vi "WPI_UtilitiesFRCAutomaticValuePublisherImpl.vi"(11 "Enable":bool=TRUE) -> ()   [LabVIEW 2025]
uses:
  <vilib>/Rock Robotics/WPI/Utilities/Refnum Registry Operation.ctl
  <vilib>/Rock Robotics/WPI/Relay/WPI_RelayValue.ctl
  <vilib>/Rock Robotics/WPI/Solenoid/WPI_SolenoidValue.ctl
  <vilib>/Rock Robotics/WPI/Solenoid/WPI_SolenoidChannel.ctl
  <vilib>/Rock Robotics/WPI/Solenoid/WPI_SolenoidSetEnum.vi
  <vilib>/Rock Robotics/WPI/Ultrasonic/WPI_SonarSRF04DigitalRefNum Registry Get.vi
  <vilib>/Rock Robotics/WPI/Ultrasonic/WPI_SonarSRF04DigitalGetRange.vi
  <vilib>/Rock Robotics/WPI/Ultrasonic/WPI_SonarSRF08_I2C_RefNum Registry Get.vi
  <vilib>/Rock Robotics/WPI/Ultrasonic/WPI_SonarSRF08_I2C_GetRange.vi
  <vilib>/Rock Robotics/WPI/Ultrasonic/WPI_SonarMB1010DigitalRefNum Registry Get.vi
  <vilib>/Rock Robotics/WPI/Ultrasonic/WPI_SonarMB1010DigitalGetRange.vi
  <vilib>/Rock Robotics/WPI/Ultrasonic/WPI_SonarMB1010AnalogRefNum Registry Get.vi
  <vilib>/Rock Robotics/WPI/Ultrasonic/WPI_SonarMB1010AnalogGetRange.vi
  <vilib>/Rock Robotics/Network Tables/NT Write Integer.vi
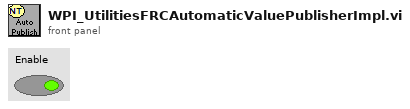
[diagram p1: front panel]
types:
  T1 = typedef "Refnum Registry Operation.ctl" = enum16{"set", "get", "delete", "get all names", "read name"}
  T2 = typedef "WPI_RelayValue.ctl" = enum16{"Off", "On", "Forward", "Reverse"}
  T3 = typedef "WPI_SolenoidChannel.ctl" = enum8{"Solenoid 0", "Solenoid 1", "Solenoid 2", "Solenoid 3", "Solenoid 4", "Solenoid 5", "Solenoid 6", "Solenoid 7", "Solenoid 8", "Solenoid 9", "Solenoid 10", "Solenoid 11", "Solenoid 12", "Solenoid 13", "Solenoid 14", "Solenoid 15", "Invalid"}
  T4 = typedef "WPI_SolenoidValue.ctl" = enum16{"Off", "On", "Forward", "Reverse"}
  T5 = enum16{"None", "XON/XOFF", "RTS/CTS", "XON/XOFF & RTS/CTS", "DTR/DSR", "XON/XOFF & DTR/DSR"}
  T6 = typedef "WPI_JoystickDevRef.ctl" = cluster{"Device":T7}
  T7 = typedef "WPI_JoystickDeviceEnum.ctl" = enum16{"USB 0", "USB 1", "USB 2", "USB 3", "USB 4", "USB 5"}
  T8 = typedef "WPI_Joystick Info.ctl" = cluster{"Device Name":string, "HID Type":T9, "XBox Type":T10, "Axes Count":i32, "Axes Types":T11[], "Button Count":i32, "POV Count":i32}
  T9 = typedef "WPI_JoystickHID Types.ctl" = enum16{"Not HID", "HID Joystick", "HID Gamepad", "HID Driving Wheel", "HID Flightstick", "HID First Person"}
  T10 = typedef "WPI_JoystickXBox Types.ctl" = enum16{"Not XBox", "XBox Unknown", "XBox Gamepad", "XBox Wheel", "XBox Arcade Stick", "XBox Flight Stick", "XBox Dance Pad", "XBox Guitar", "XBox Drum Kit", "XBox Arcade Pad"}
  T11 = typedef "WPI_JoystickAxis Types.ctl" = enum16{"X Axis", "Y Axis", "Z Axis", "RxAxis", "RyAxis", "RzAxis", "Slider", "POV", "None", "L X Axis", "L Y Axis", "L Trigger", "R Trigger", "R X Axis", "R Y Axis"}
  T12 = typedef "WPI_MotorControlDeviceRef.ctl" = cluster{"DeviceStatus":errorcluster, "Type":T13, "PWM":cluster{"PWM Channel":T14, "DeadBand":T15}, "CAN":cluster{"Device Number":u8, "SetOutput VI Ref":variant, "GetOutput VI Ref":variant, "Enable VI Ref":variant, "Disable VI Ref":variant, "Data":variant}, "Invert":bool, "DIO PWM":cluster{"PWM \"Enable\" Channel":T14, "DIOChannel":T16, "PWM Rate":dbl}}
  T13 = typedef "WPI_MotorControlType.ctl" = enum16{"PWM", "CAN", "DIO PWM"}
  T14 = typedef "FPGA_DIOPWMChannel.ctl" = enum8{"PWM 0", "PWM 1", "PWM 2", "PWM 3", "PWM 4", "PWM 5", "PWM 6", "PWM 7", "PWM 8", "PWM 9", "PWM MXP 0", "PWM MXP 1", "PWM MXP 2", "PWM MXP 3", "PWM MXP 4", "PWM MXP 5", "PWM MXP 6", "PWM MXP 7", "PWM MXP 8", "PWM MXP 9", "Invalid"}
  T15 = typedef "WPI_PWMDeadband.ctl" = cluster{"Name":string, "maxPositivePwm":i32, "minPositivePwm":i32, "centerPwm":i32, "maxNegativePwm":i32, "minNegativePwm":i32, "angularRange":u16}
  T16 = typedef "FPGA_DIOChannel.ctl" = enum8{"DIO 0", "DIO 1", "DIO 2", "DIO 3", "DIO 4", "DIO 5", "DIO 6", "DIO 7", "DIO 8", "DIO 9", "DIO MXP 0", "DIO MXP 1", "DIO MXP 2", "DIO MXP 3", "DIO MXP 4", "DIO MXP 5", "DIO MXP 6", "DIO MXP 7", "DIO MXP 8", "DIO MXP 9", "DIO MXP 10", "DIO MXP 11", "DIO MXP 12", "DIO MXP 13", "DIO MXP 14", "DIO MXP 15", "SPI Port CS1", "SPI Port CS2", "SPI Port CS3", "SPI Port MISO", "SPI Port MOSI", "Invalid"}
  T17 = typedef "WPI_ServoDeviceRef.ctl" = cluster{"DeviceStatus":errorcluster, "PWM Channel":T14, "DeadBand":T15}
  T18 = typedef "WPI_RelayDevRef.ctl" = cluster{"DevStatus":errorcluster, "Relay Channel":T19, "Relay Direction":T20}
  T19 = typedef "FPGA_DIORelayChannel.ctl" = enum8{"Relay 0", "Relay 1", "Relay 2", "Relay 3", "Invalid"}
  T20 = typedef "WPI_RelayDirection.ctl" = enum16{"Both directions", "Forward only", "Reverse only"}
  T21 = typedef "WPI_CompressorDevRef.ctl" = cluster{"DevStatus":errorcluster, "Pneumatics Control Module":u8}
  T22 = typedef "WPI_SolenoidDevRef.ctl" = cluster{"DevStatus":errorcluster, "Pneumatics Control Module":u8, "Forward Solenoid Channel":T3, "Reverse Solenoid Channel":T3}
  T23 = typedef "WPI_AccelerometerDevRef.ctl" = cluster{"DevStatus":errorcluster, "Scaling":T24, "Analog Channels":T25, "I2C Bus":T27, "SPI Bus":T28, "Accel Range":T29, "ADXL Axes":T30, "Handle":i32, "Device Address":u8, "Accel Type":enum16{"Analog", "ADXL345 I2C", "ADXL345 SPI", "Internal", "ADXL362 SPI"}}
  T24 = typedef "WPI_AccelerometerScaling.ctl" = cluster{"Gain (VoltsPerG)":dbl, "Center Voltage":dbl}
  T25 = typedef "WPI_AccelerometerAnalogChannels.ctl" = cluster{"X-Axis":T26, "Y-Axis":T26, "Z-Axis":T26}
  T26 = typedef "FPGA_AIChannel.ctl" = enum8{"AI 0", "AI 1", "AI 2", "AI 3", "AI MXP 0", "AI MXP 1", "AI MXP 2", "AI MXP 3", "Invalid"}
  T27 = typedef "i2c_bus.ctl" = enum16{"I2C On-Board", "I2C MXP", "Invalid"}
  T28 = typedef "spi_bus.ctl" = enum16{"SPI On-Board, CS0", "SPI On-Board, CS1", "SPI On-Board, CS2", "SPI On-Board, CS3", "SPI MXP", "Invalid"}
  T29 = typedef "ADXL345 Range.ctl" = u8
  T30 = typedef "WPI_AccelerometerADXL345 Axes.ctl" = cluster{"X-Axis":bool, "Y-Axis":bool, "Z-Axis":bool}
  T31 = cluster{"X-Axis":dbl, "Y-Axis":dbl, "Z-Axis":dbl}
  T32 = typedef "WPI_CounterDevRef.ctl" = cluster{"DevStatus":errorcluster, "CntIndex":T33}
  T33 = typedef "FPGA_CounterCtrSystemIndex.ctl" = enum8{"Ctr 0", "Ctr 1", "Ctr 2", "Ctr 3", "Ctr 4", "Ctr 5", "Ctr 6", "Ctr 7", "Invalid"}
  T34 = typedef "WPI_GyroDevRef.ctl" = cluster{"DevStatus":errorcluster, "Analog Channel":T26, "Gain (VoltsPerDegree/Second)":dbl, "Gyro Type":enum16{"Analog", "XRS450"}, "Handle":i32, "SPI Bus":T28, "Device Found":bool, "Sample Rate":dbl, "Calibrate On Open":bool, "Offset":dbl}
  T35 = typedef "WPI_UltrasonicDeviceRef.ctl" = cluster{"DevStatus":errorcluster, "Ping Channel":T16, "Echo Channel":T16, "CntIndex":T33}
  T36 = typedef "WPI_SonarSRF08_I2C_DeviceRef.ctl" = cluster{"I2CDevRef":T37}
  T37 = typedef "WPI_I2CDevRef.ctl" = cluster{"DevStatus":errorcluster, "Device Address":u8, "Handle":i32, "I2C Bus":T27}
  T38 = typedef "WPI_SonarMB1010DigitalDeviceRef.ctl" = cluster{"CounterDevRef":T32, "Scaling factor (s/in)":dbl}
  T39 = typedef "WPI_SonarMB1010AnalogDeviceRef.ctl" = cluster{"AIDeviceRef":T40, "Scaling factor (V/in)":dbl, "Average Bits":u8}
  T40 = typedef "WPI_AnalogChannelDevRef.ctl" = cluster{"DevStatus":errorcluster, "Analog Channel":T26}
  T41 = typedef "WPI_DigitalInputDevRef.ctl" = cluster{"DevStatus":errorcluster, "DIO Channel":T16}
  T42 = typedef "WPI_SwitchDevRef.ctl" = cluster{"DevStatus":errorcluster, "DIO Channel":T16, "CntIndex":T33, "Normally Closed":bool}
  T43 = typedef "WPI_EncoderDevRef.ctl" = cluster{"DevStatus":errorcluster, "EncoderIndex":T44, "CounterIndex":T33, "DistancePerCount":dbl, "Decoding Type":T45}
  T44 = typedef "FPGA_EncoderIdx.ctl" = enum8{"Enc 0", "Enc 1", "Enc 2", "Enc 3", "Enc 4", "Enc 5", "Enc 6", "Enc 7", "Invalid"}
  T45 = typedef "WPI_EncoderType.ctl" = enum16{"1x", "2x", "4x"}
  T46 = typedef "WPI_DigitalOutputDevRef.ctl" = cluster{"DIO Channel":T16, "DevStatus":errorcluster}
  T47 = typedef "WPI_AOChannelDevRef.ctl" = cluster{"DevStatus":errorcluster, "AO Channel":T48}
  T48 = typedef "WPI_AnalogOutputChannel.ctl" = enum8{"AO MXP 0", "AO MXP 1", "Invalid"}
  T49 = typedef "WPI_PWMDeviceRef.ctl" = cluster{"DeviceStatus":errorcluster, "PWM Channel":T14}
  T50 = typedef "WPI_PotentiometerDevRef.ctl" = cluster{"DevStatus":errorcluster, "Analog Channel":T26, "Invert Output":bool}
  T51 = typedef "WPI_CameraDevRef.ctl" = cluster{"Camera Address":string, "CameraStatus":errorcluster}
  T52 = typedef "WPI_SerialPortRef.ctl" = cluster{"DevStatus":errorcluster, "Serial Port Name":refnum<visa-resource-name>}
  T53 = typedef "WPI_SPIDevRef.ctl" = cluster{"DevStatus":errorcluster, "Handle":i32, "SPI Bus":T28}
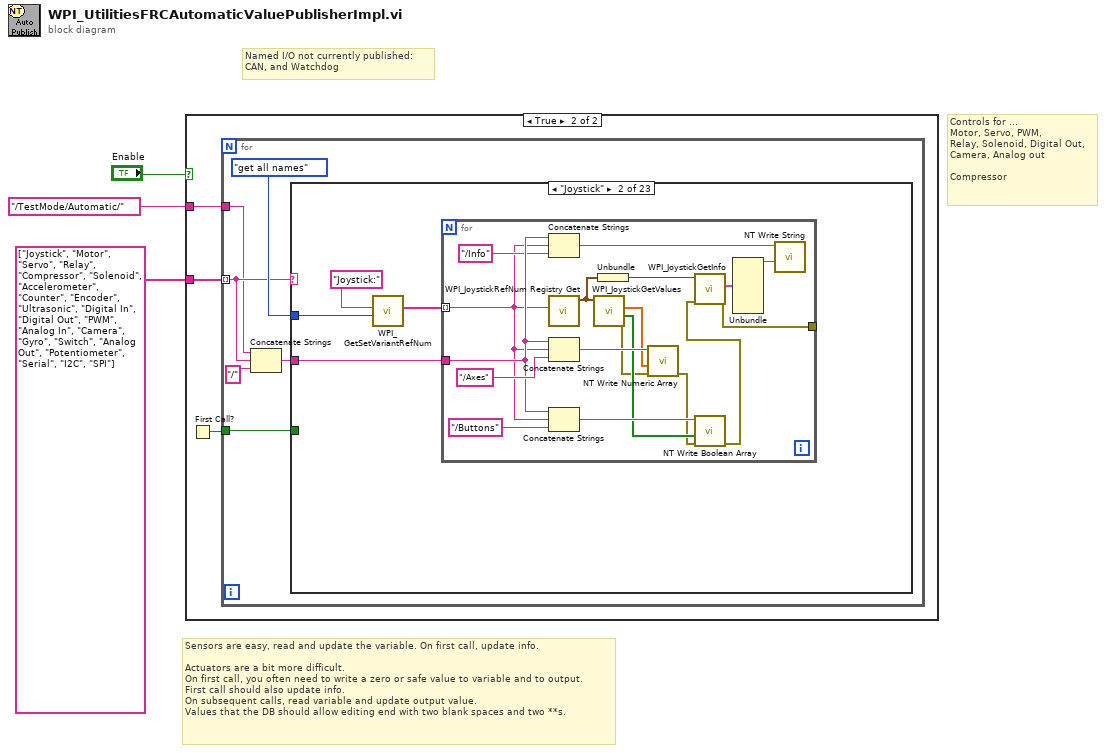
[diagram p0: block diagram]
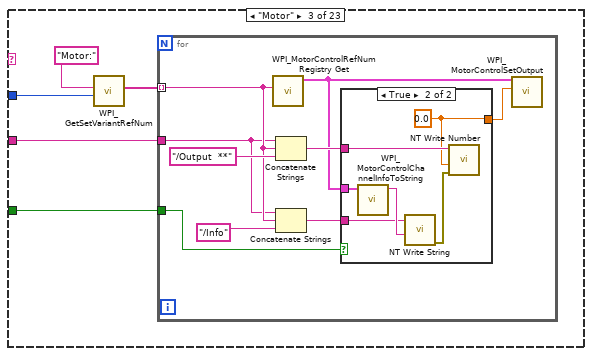
[diagram p4: hidden frame]
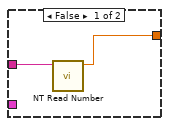
[diagram p5: hidden frame]
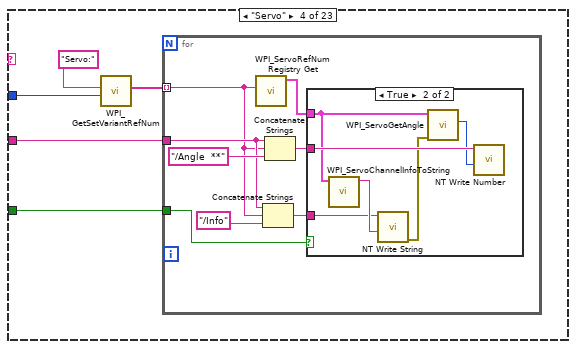
[diagram p6: hidden frame]
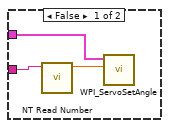
[diagram p7: hidden frame]
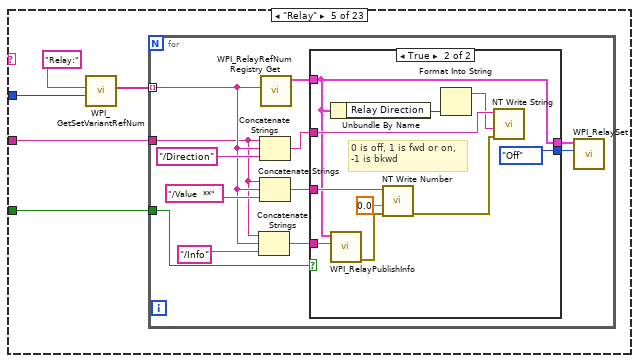
[diagram p8: hidden frame]
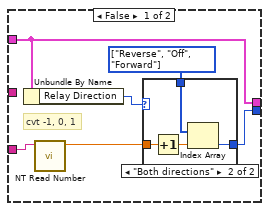
[diagram p9: hidden frame]
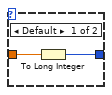
[diagram p10: hidden frame]
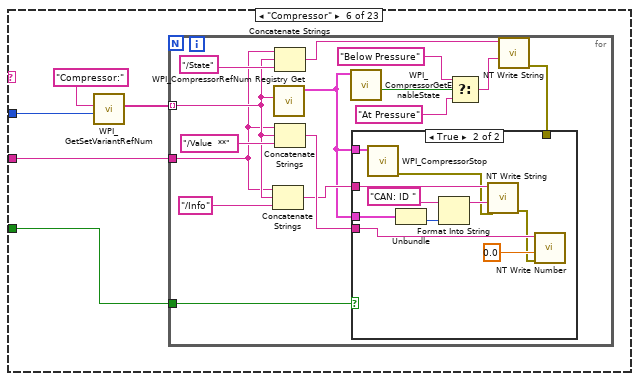
[diagram p11: hidden frame]
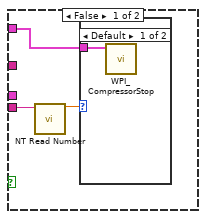
[diagram p12: hidden frame]
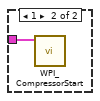
[diagram p13: hidden frame]
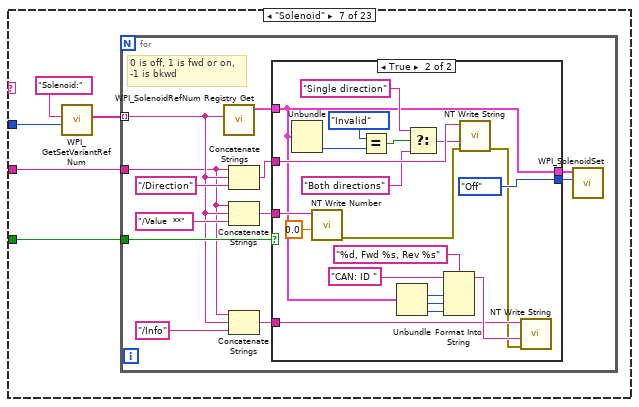
[diagram p14: hidden frame]
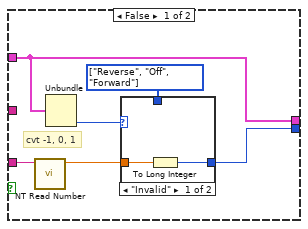
[diagram p15: hidden frame]
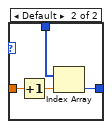
[diagram p16: hidden frame]
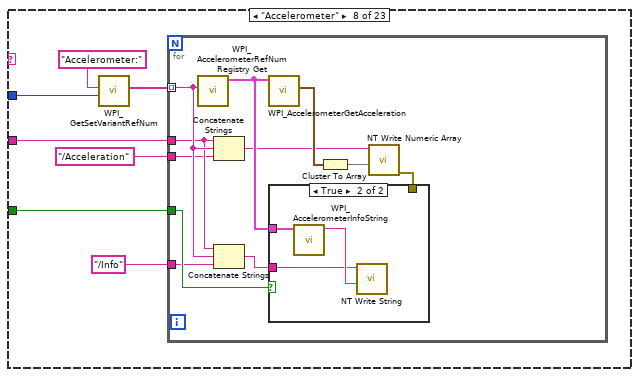
[diagram p17: hidden frame]
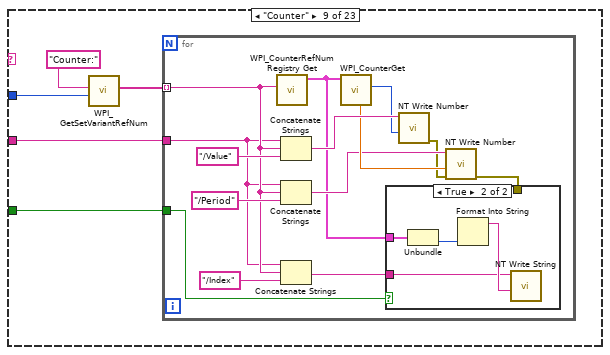
[diagram p19: hidden frame]
diagram:
  # "Controls for ...\nMotor, Servo, PWM,\nRelay, Solenoid, Digital Out,\nCamera, Analog out\n\nCompressor"
  # "Named I/O not currently published:\nCAN, and Watchdog"
  # "Sensors are easy, read and update the variable. On first call, update info.\n\nActuators are a bit more difficult. \nOn first call, you often need to write a zero or safe value to variable and to output.\nFirst call should also update info.\nOn subsequent calls, read variable and update output value.\nValues that the DB should allow editing end with two blank spaces and two **s."
  n1 = case shown="True" "Enable" {
    tunnel: string[] ["Joystick", "Motor", "Servo", "Relay", "Compressor", "Solenoid", "Accelerometer", "Counter", "Encoder", "Ultrasonic", "Digital In", "Digital Out", "PWM", "Analog In", "Camera", "Gyro", "Switch", "Analog Out", "Potentiometer", "Serial", "I2C", "SPI"] -> [_ w6]
    tunnel: "/TestMode/Automatic/" -> [_ w4]
    frame False {
    }
    frame True {
      n2 = First Call?() -> (First Call?: T/F=w5:bool)
      n3 = for {
        tunnel: w6 -> [w10] mode=indexing
        tunnel: w5 -> [w11]
        tunnel: w4 -> [w9]
        n4 = Concatenate Strings(w9, w10, "/") -> (w7:string)
        n5 = case shown="\"Joystick\"" w10 {
          tunnel: Refnum_Registry_Operation."get all names" ("menu") -> [_ w14 w36 w57 w79 w119 w153 w204 w223 w246 w271 w358 w375 w400 w426 w453 w479 w503 w523 w547 w569 w602 w618]
          tunnel: w11 -> [_ _ w39 w61 w83 w122 w157 w208 w227 w250 w273 w362 w379 w404 w430 w457 w483 w507 w527 w551 w568 w601 w617]
          tunnel: w7 -> [_ w16 w38 w60 w82 w121 w156 w207 w226 w249 w272 w361 w378 w403 w429 w456 w482 w506 w526 w550 w570 w603 w619]
          frame Default {
            # "Unsupported I/O type"
          }
          frame "Joystick" {
            n6 = call <vilib>:"WPI_GetSetVariantRefNum.vi"("Operation"=w14, "refnum name"="Joystick:") -> ("names"=w15:string[])  [unwired: 7 in, 2 out]
            n7 = for {
              tunnel: w15 -> [w23] mode=indexing
              tunnel: w16 -> [w25]
              tunnel: [w19] -> _
              n8 = Concatenate Strings(w25, w23, "/Info") -> (w18:string)
              n9 = call <vilib>:"WPI_JoystickRefNum Registry Get.vi"("refnum name"=w23) -> ("JoystickDevRef"=w28:T6)  [unwired: 9 in, 1 out]
              n10 = Concatenate Strings(w25, w23, "/Axes") -> (w31:string)
              n11 = Concatenate Strings(w25, w23, "/Buttons") -> (w33:string)
              n12 = call <vilib>:"WPI_JoystickGetValues.vi"("JoystickDevRef"=w28) -> ("error out"=w20:errorcluster, "Buttons"=w29:bool[], "Axes"=w30:dbl[])  [unwired: 6 in, 2 out]
              n13 = Unbundle(w28) -> ("Device"=w27:T7)
              n14 = call <vilib>:"NT Write Numeric Array.vi"("error in"=w20, "value"=w30, "name"=w31) -> ("error out"=w22:errorcluster)  [unwired: 8 in]
              n15 = call <vilib>:"NT Write Boolean Array.vi"("error in"=w22, "value"=w29, "name"=w33) -> ("error out"=w21:errorcluster)  [unwired: 8 in]
              n16 = call <vilib>:"WPI_JoystickGetInfo.vi"("error in (no error)"=w21, "JoystickDevice"=w27) -> ("error out"=w19:errorcluster, "Joystick Info"=w26:T8)  [unwired: 8 in]
              n17 = Unbundle(w26) -> ("Device Name"=w17:string)  [unwired: 6 out]
              n18 = call <vilib>:"NT Write String.vi"("value"=w17, "name"=w18) -> ()  [unwired: 9 in, 1 out]
            }
          }
          frame "Motor" {
            n19 = call <vilib>:"WPI_GetSetVariantRefNum.vi"("Operation"=w36, "refnum name"="Motor:") -> ("names"=w35:string[])  [unwired: 7 in, 2 out]
            n20 = for {
              tunnel: w35 -> [w43] mode=indexing
              tunnel: w39 -> [w45]
              tunnel: w38 -> [w42]
              n21 = call <vilib>:"WPI_MotorControlRefNum Registry Get.vi"("refnum name"=w43) -> ("MotorControlDevRef"=w41:T12)  [unwired: 9 in, 1 out]
              n22 = Concatenate Strings(w42, w43, "/Output  **") -> (w47:string)
              n23 = Concatenate Strings(w42, w43, "/Info") -> (w40:string)
              n24 = case shown="True" w45 {
                tunnel: w47 -> [w50 w56]
                tunnel: [w49 w55] -> w46
                tunnel: w41 -> [_ w53]
                tunnel: w40 -> [_ w52]
                frame False {
                  n25 = call <vilib>:"NT Read Number.vi"("name"=w50) -> ("value"=w49:dbl)  [unwired: 8 in, 2 out]
                }
                frame True {
                  w55 = 0.0
                  n26 = call <vilib>:"WPI_MotorControlChannelInfoToString.vi"("MotorControlDevRef"=w53) -> ("String"=w54:string)  [unwired: 10 in]
                  n27 = call <vilib>:"NT Write String.vi"("value"=w54, "name"=w52) -> ("error out"=w51:errorcluster)  [unwired: 9 in]
                  n28 = call <vilib>:"NT Write Number.vi"("error in"=w51, "value"=w55, "name"=w56) -> ()  [unwired: 8 in, 1 out]
                }
              }
              n29 = call <vilib>:"WPI_MotorControlSetOutput.vi"("Output"=w46, "MotorControlDevRef"=w41) -> ()  [unwired: 7 in, 3 out]
            }
          }
          frame "Servo" {
            n30 = call <vilib>:"WPI_GetSetVariantRefNum.vi"("Operation"=w57, "refnum name"="Servo:") -> ("names"=w58:string[])  [unwired: 7 in, 2 out]
            n31 = for {
              tunnel: w58 -> [w62] mode=indexing
              tunnel: w61 -> [w67]
              tunnel: w60 -> [w64]
              n32 = call <vilib>:"WPI_ServoRefNum Registry Get.vi"("refnum name"=w62) -> ("ServoDeviceRef"=w66:T17)  [unwired: 9 in, 1 out]
              n33 = Concatenate Strings(w64, w62, "/Info") -> (w63:string)
              n34 = Concatenate Strings(w64, w62, "/Angle  **") -> (w68:string)
              n35 = case shown="True" w67 {
                tunnel: w68 -> [w72 w78]
                tunnel: w66 -> [w70 w76]
                tunnel: w63 -> [_ w74]
                frame False {
                  n36 = call <vilib>:"NT Read Number.vi"("name"=w72) -> ("value"=w71:dbl)  [unwired: 8 in, 2 out]
                  n37 = call <vilib>:"WPI_ServoSetAngle.vi"("Angle"=w71, "ServoDeviceRef"=w70) -> ()  [unwired: 8 in, 2 out]
                }
                frame True {
                  n38 = call <vilib>:"WPI_ServoChannelInfoToString.vi"("ServoDeviceRef"=w76) -> ("String"=w75:string)  [unwired: 10 in]
                  n39 = call <vilib>:"NT Write String.vi"("value"=w75, "name"=w74) -> ("error out"=w73:errorcluster)  [unwired: 9 in]
                  n40 = call <vilib>:"WPI_ServoGetAngle.vi"("ServoDeviceRef"=w76, "error in (no error)"=w73) -> ("Angle"=w77:u16)  [unwired: 6 in, 2 out]
                  n41 = call <vilib>:"NT Write Number.vi"("value"=w77, "name"=w78) -> ()  [unwired: 9 in, 1 out]
                }
              }
            }
          }
          frame "Relay" {
            n42 = call <vilib>:"WPI_GetSetVariantRefNum.vi"("Operation"=w79, "refnum name"="Relay:") -> ("names"=w80:string[])  [unwired: 7 in, 2 out]
            n43 = for {
              tunnel: w80 -> [w86] mode=indexing
              tunnel: w83 -> [w93]
              tunnel: w82 -> [w85]
              n44 = Concatenate Strings(w85, w86, "/Info") -> (w84:string)
              n45 = Concatenate Strings(w85, w86, "/Direction") -> (w94:string)
              n46 = Concatenate Strings(w85, w86, "/Value  **") -> (w90:string)
              n47 = call <vilib>:"WPI_RelayRefNum Registry Get.vi"("refnum name"=w86) -> ("RelayDevRef"=w92:T18)  [unwired: 9 in, 1 out]
              n48 = case shown="True" w93 {
                tunnel: w94 -> [_ w117]
                tunnel: w92 -> [w96 w111]
                tunnel: w90 -> [w101 w114]
                tunnel: [w96 w111] -> w89
                tunnel: [w98 WPI_RelayValue."Off" ("RelayValue")] -> w88
                tunnel: w84 -> [_ w112]
                frame False {
                  w99 = T2[] [enum."Reverse", enum."Off", enum."Forward"] items=["Off", "On", "Forward", "Reverse"]
                  # "cvt -1, 0, 1"
                  n49 = Unbundle By Name(w96) -> ("Relay Direction"=w97:T20)
                  n50 = call <vilib>:"NT Read Number.vi"("name"=w101) -> ("value"=w100:dbl)  [unwired: 8 in, 2 out]
                  n51 = case shown="\"Both directions\"" w97 {
                    tunnel: w100 -> [w103 w107]
                    tunnel: w99 -> [_ w105]
                    tunnel: [w102 w104] -> w98
                    frame Default {
                      n52 = To Long Integer(number=w103) -> (32bit integer=w102:i32)
                    }
                    frame "Both directions" {
                      n53 = Increment(x=w107) -> (x+1=w106:dbl)
                      n54 = Index Array(array=w105, index=w106) -> (element=w104:T2)
                    }
                  }
                }
                frame True {
                  # "0 is off, 1 is fwd or on,\n-1 is bkwd"
                  n55 = Unbundle By Name(w111) -> ("Relay Direction"=w110:T20)
                  n56 = call <vilib>:"WPI_RelayPublishInfo.vi"("Name"=w112, "RelayDevRef"=w111) -> ("error out"=w109:errorcluster)  [unwired: 9 in]
                  n57 = call <vilib>:"NT Write Number.vi"("error in"=w109, "value"=0.0 ("Numeric"), "name"=w114) -> ("error out"=w108:errorcluster)  [unwired: 8 in]
                  n58 = Format Into String(w110) -> (resulting string=w116:string)  [unwired: 3 in, 1 out]
                  n59 = call <vilib>:"NT Write String.vi"("error in"=w108, "value"=w116, "name"=w117) -> ()  [unwired: 8 in, 1 out]
                }
              }
              n60 = call <vilib>:"WPI_RelaySet.vi"("RelayValue"=w88, "RelayDevRef"=w89) -> ()  [unwired: 8 in, 2 out]
            }
          }
          frame "Compressor" {
            n61 = call <vilib>:"WPI_GetSetVariantRefNum.vi"("Operation"=w119, "refnum name"="Compressor:") -> ("names"=w118:string[])  [unwired: 7 in, 2 out]
            n62 = for {
              tunnel: w118 -> [w131] mode=indexing
              tunnel: w122 -> [w136]
              tunnel: w121 -> [w130]
              n63 = Concatenate Strings(w130, w131, "/Info") -> (w129:string)
              n64 = call <vilib>:"WPI_CompressorRefNum Registry Get.vi"("refnum name"=w131) -> ("CompressorDevRef"=w128:T21)  [unwired: 9 in, 1 out]
              n65 = Concatenate Strings(w130, w131, "/State") -> (w134:string)
              n66 = Concatenate Strings(w130, w131, "/Value  **") -> (w132:string)
              n67 = call <vilib>:"WPI_CompressorGetEnableState.vi"("CompressorDevRef"=w128) -> ("Compressor Running"=w127:bool)  [unwired: 4 in, 6 out]
              n68 = Select(t="Below Pressure", s=w127, f="At Pressure") -> (s? t:f=w124:string)
              n69 = call <vilib>:"NT Write String.vi"("value"=w124, "name"=w134) -> ("error out"=w123:errorcluster)  [unwired: 9 in]
              n70 = case shown="True" w136 {
                tunnel: w128 -> [_ w149]
                tunnel: w128 -> [w140 w150]
                tunnel: w132 -> [w139 w152]
                tunnel: w129 -> [_ w146]
                tunnel: w123 -> [_ _]
                frame False {
                  n71 = call <vilib>:"NT Read Number.vi"("name"=w139) -> ("value"=w138:dbl)  [unwired: 8 in, 2 out]
                  n72 = case shown="Default" w138 {
                    tunnel: w140 -> [w141 w142]
                    frame Default {
                      n73 = call <vilib>:"WPI_CompressorStop.vi"("CompressorDevRef"=w141) -> ()  [unwired: 9 in, 2 out]
                    }
                    frame 1 {
                      n74 = call <vilib>:"WPI_CompressorStart.vi"("CompressorDevRef"=w142) -> ()  [unwired: 9 in, 2 out]
                    }
                  }
                }
                frame True {
                  n75 = call <vilib>:"WPI_CompressorStop.vi"("CompressorDevRef"=w150) -> ("error out"=w144:errorcluster)  [unwired: 9 in, 1 out]
                  n76 = Unbundle(w149) -> ("Pneumatics Control Module"=w148:u8)  [unwired: 1 out]
                  n77 = Format Into String(initial string="CAN: ID ", w148) -> (resulting string=w147:string)  [unwired: 2 in, 1 out]
                  n78 = call <vilib>:"NT Write String.vi"("error in"=w144, "value"=w147, "name"=w146) -> ("error out"=w143:errorcluster)  [unwired: 8 in]
                  n79 = call <vilib>:"NT Write Number.vi"("error in"=w143, "value"=0.0 ("Numeric"), "name"=w152) -> ()  [unwired: 8 in, 1 out]
                }
              }
            }
          }
          frame "Solenoid" {
            n80 = call <vilib>:"WPI_GetSetVariantRefNum.vi"("Operation"=w153, "refnum name"="Solenoid:") -> ("names"=w154:string[])  [unwired: 7 in, 2 out]
            n81 = for {
              tunnel: w154 -> [w160] mode=indexing
              tunnel: w157 -> [w165]
              tunnel: w156 -> [w159]
              # "0 is off, 1 is fwd or on,\n-1 is bkwd"
              n82 = call <vilib>:"WPI_SolenoidRefNum Registry Get.vi"("refnum name"=w160) -> ("SolenoidDevRef"=w162:T22)  [unwired: 9 in, 1 out]
              n83 = Concatenate Strings(w159, w160, "/Direction") -> (w168:string)
              n84 = Concatenate Strings(w159, w160, "/Value  **") -> (w163:string)
              n85 = Concatenate Strings(w159, w160, "/Info") -> (w158:string)
              n86 = case shown="True" w165 {
                tunnel: w168 -> [_ w201]
                tunnel: w162 -> [w172 w186]
                tunnel: w163 -> [w175 w199]
                tunnel: [w172 w186] -> w167
                tunnel: [w171 WPI_SolenoidValue."Off" ("Relay Value")] -> w166
                tunnel: w158 -> [_ w188]
                frame False {
                  w173 = T4[] [enum."Reverse", enum."Off", enum."Forward"] items=["Off", "On", "Forward", "Reverse"]
                  # "cvt -1, 0, 1"
                  n87 = call <vilib>:"NT Read Number.vi"("name"=w175) -> ("value"=w174:dbl)  [unwired: 8 in, 2 out]
                  n88 = Unbundle(w172) -> ("Reverse Solenoid Channel"=w170:T3)  [unwired: 3 out]
                  n89 = case shown="\"Invalid\"" w170 {
                    tunnel: w174 -> [w177 w181]
                    tunnel: w173 -> [_ w179]
                    tunnel: [w176 w178] -> w171
                    frame "Invalid" {
                      n90 = To Long Integer(number=w177) -> (32bit integer=w176:i32)
                    }
                    frame Default {
                      n91 = Increment(x=w181) -> (x+1=w180:dbl)
                      n92 = Index Array(array=w179, index=w180) -> (element=w178:T4)
                    }
                  }
                }
                frame True {
                  n93 = Unbundle(w186) -> ("Reverse Solenoid Channel"=w197:T3)  [unwired: 3 out]
                  n94 = call <vilib>:"NT Write Number.vi"("value"=0.0 ("Numeric"), "name"=w199) -> ("error out"=w183:errorcluster)  [unwired: 9 in]
                  n95 = Equal?(x=WPI_SolenoidChannel."Invalid" ("Reverse Solenoid Channel"), y=w197) -> (x = y?=w196:bool)
                  n96 = Unbundle(w186) -> ("Pneumatics Control Module"=w189:u8, "Forward Solenoid Channel"=w190:T3, "Reverse Solenoid Channel"=w185:T3)  [unwired: 1 out]
                  n97 = Select(t="Single direction", s=w196, f="Both directions") -> (s? t:f=w192:string)
                  n98 = Format Into String(format string="%d, Fwd %s, Rev %s", initial string="CAN: ID " ("format string"), w189, w190, w185) -> (resulting string=w191:string)  [unwired: 1 in, 1 out]
                  n99 = call <vilib>:"NT Write String.vi"("error in"=w183, "value"=w192, "name"=w201) -> ("error out"=w182:errorcluster)  [unwired: 8 in]
                  n100 = call <vilib>:"NT Write String.vi"("error in"=w182, "value"=w191, "name"=w188) -> ()  [unwired: 8 in, 1 out]
                }
              }
              n101 = call-poly <vilib>:"WPI_SolenoidSet.vi"("Value"=w166, "SolenoidDevRef"=w167) -> ()  [unwired: 8 in, 2 out]
            }
          }
          frame "Accelerometer" {
            n102 = call <vilib>:"WPI_GetSetVariantRefNum.vi"("Operation"=w204, "refnum name"="Accelerometer:") -> ("names"=w205:string[])  [unwired: 7 in, 2 out]
            n103 = for {
              tunnel: w205 -> [w218] mode=indexing
              tunnel: w208 -> [w216]
              tunnel: w207 -> [w217]
              tunnel: "/Acceleration" -> [w213]
              tunnel: "/Info" -> [w212]
              n104 = call <vilib>:"WPI_AccelerometerRefNum Registry Get.vi"("refnum name"=w218) -> ("AccelerometerDevRef"=w215:T23)  [unwired: 9 in, 1 out]
              n105 = Concatenate Strings(w217, w218, w213) -> (w211:string)
              n106 = Concatenate Strings(w217, w218, w212) -> (w214:string)
              n107 = call <vilib>:"WPI_AccelerometerGetAcceleration.vi"("AccelerometerDevRef"=w215) -> ("Accelerations"=w219:T31)  [unwired: 8 in, 2 out]
              n108 = Cluster To Array(cluster=w219) -> (array=w210:dbl[])
              n109 = call <vilib>:"NT Write Numeric Array.vi"("value"=w210, "name"=w211) -> ("error out"=w209:errorcluster)  [unwired: 9 in]
              n110 = case shown="True" w216 {
                tunnel: w214 -> [_ w220]
                tunnel: w215 -> [_ w222]
                tunnel: w209 -> [_ _]
                frame False {
                }
                frame True {
                  n111 = call <vilib>:"WPI_AccelerometerInfoString.vi"("AccelerometerDevRef"=w222) -> ("String"=w221:string)  [unwired: 10 in]
                  n112 = call <vilib>:"NT Write String.vi"("value"=w221, "name"=w220) -> ()  [unwired: 9 in, 1 out]
                }
              }
            }
          }
          frame "Counter" {
            n113 = call <vilib>:"WPI_GetSetVariantRefNum.vi"("Operation"=w223, "refnum name"="Counter:") -> ("names"=w224:string[])  [unwired: 7 in, 2 out]
            n114 = for {
              tunnel: w224 -> [w232] mode=indexing
              tunnel: w227 -> [w230]
              tunnel: w226 -> [w231]
              n115 = call <vilib>:"WPI_CounterRefNum Registry Get.vi"("refnum name"=w232) -> ("CounterDevRef"=w235:T32)  [unwired: 9 in, 1 out]
              n116 = Concatenate Strings(w231, w232, "/Value") -> (w240:string)
              n117 = Concatenate Strings(w231, w232, "/Period") -> (w236:string)
              n118 = Concatenate Strings(w231, w232, "/Index") -> (w233:string)
              n119 = call <vilib>:"WPI_CounterGet.vi"("CounterDevRef in"=w235) -> ("Value"=w239:i32, "Period (sec)"=w238:dbl)  [unwired: 5 in, 4 out]
              n120 = call <vilib>:"NT Write Number.vi"("value"=w239, "name"=w240) -> ("error out"=w229:errorcluster)  [unwired: 9 in]
              n121 = call <vilib>:"NT Write Number.vi"("error in"=w229, "value"=w238, "name"=w236) -> ("error out"=w228:errorcluster)  [unwired: 8 in]
              n122 = case shown="True" w230 {
                tunnel: w233 -> [_ w242]
                tunnel: w235 -> [_ w245]
                tunnel: w228 -> [_ _]
                frame False {
                }
                frame True {
                  n123 = Unbundle(w245) -> ("CntIndex"=w244:T33)  [unwired: 1 out]
                  n124 = Format Into String(w244) -> (resulting string=w243:string)  [unwired: 3 in, 1 out]
                  n125 = call <vilib>:"NT Write String.vi"("value"=w243, "name"=w242) -> ()  [unwired: 9 in, 1 out]
                }
              }
            }
          }
          frame "Gyro" {
            n126 = call <vilib>:"WPI_GetSetVariantRefNum.vi"("Operation"=w246, "refnum name"="Gyro:") -> ("names"=w247:string[])  [unwired: 7 in, 2 out]
            n127 = for {
              tunnel: w247 -> [w257] mode=indexing
              tunnel: w250 -> [w254]
              tunnel: w249 -> [w256]
              n128 = call <vilib>:"WPI_GyroRefNum Registry Get.vi"("refnum name"=w257) -> ("GyroDevRef"=w253:T34)  [unwired: 9 in, 1 out]
              n129 = Concatenate Strings(w256, w257, "/Angle") -> (w263:string)
              n130 = Concatenate Strings(w256, w257, "/Rate") -> (w261:string)
              n131 = Concatenate Strings(w256, w257, "/Info") -> (w255:string)
              n132 = call <vilib>:"WPI_GyroGetAngle.vi"("GyroDevRef"=w253) -> ("Angular Rate"=w259:dbl, "Angle"=w260:dbl)  [unwired: 6 in, 3 out]
              n133 = call <vilib>:"NT Write Number.vi"("value"=w260, "name"=w263) -> ("error out"=w252:errorcluster)  [unwired: 9 in]
              n134 = call <vilib>:"NT Write Number.vi"("error in"=w252, "value"=w259, "name"=w261) -> ("error out"=w251:errorcluster)  [unwired: 8 in]
              n135 = case shown="True" w254 {
                tunnel: w255 -> [_ w267]
                tunnel: w253 -> [_ w266]
                tunnel: w251 -> [_ _]
                frame False {
                }
                frame True {
                  n136 = Unbundle By Name(w266) -> ("Analog Channel"=w265:T26)
                  n137 = Format Into String(format string="%s", w265) -> (resulting string=w268:string)  [unwired: 2 in, 1 out]
                  n138 = call <vilib>:"NT Write String.vi"("value"=w268, "name"=w267) -> ()  [unwired: 9 in, 1 out]
                }
              }
            }
          }
          frame "Ultrasonic" {
            n139 = for {
              tunnel: w273 -> [w281]
              tunnel: w272 -> [w280]
              tunnel: w271 -> [w278]
              tunnel: string[] ["Ultrasonic:SRF04Dig:", "Ultrasonic:SRF08:", "Ultrasonic:M1010Dig:", "Ultrasonic:M1010An:"] -> [w275] mode=indexing
              i -> [w274]
              n140 = call <vilib>:"WPI_GetSetVariantRefNum.vi"("Operation"=w278, "refnum name"=w275) -> ("names"=w279:string[])  [unwired: 7 in, 2 out]
              n141 = for {
                tunnel: w279 -> [w287] mode=indexing
                tunnel: w281 -> [w285]
                tunnel: w280 -> [w286]
                tunnel: "/Info" -> [w284]
                tunnel: "/Distance" -> [w283]
                tunnel: w274 -> [w282]
                n142 = case shown="0" w282 {
                  tunnel: w287 -> [_ w295 w315 w332 w349]
                  tunnel: w286 -> [_ w294 w314 w331 w348]
                  tunnel: w285 -> [_ w292 w313 w330 w347]
                  tunnel: w284 -> [_ w289 w312 w329 w346]
                  tunnel: w283 -> [_ w288 w311 w328 w345]
                  frame Default {
                  }
                  frame 0 {
                    n143 = call-poly <vilib>:"WPI_UltrasonicRefNum Registry Get.vi"("refnum name"=w295) -> ("SonarSRF04DevRef"=w291:T35)  [unwired: 9 in, 1 out]
                    n144 = Concatenate Strings(w294, w295, w288) -> (w297:string)
                    n145 = Concatenate Strings(w294, w295, w289) -> (w293:string)
                    n146 = call-poly <vilib>:"WPI_UltrasonicGetRange.vi"("UltrasonicDevRef"=w291) -> ("Distance"=w296:dbl)  [unwired: 8 in, 2 out]
                    n147 = call <vilib>:"NT Write Number.vi"("value"=w296, "name"=w297) -> ("error out"=w290:errorcluster)  [unwired: 9 in]
                    n148 = case shown="True" w292 {
                      tunnel: w293 -> [_ w302]
                      tunnel: w291 -> [_ w301]
                      tunnel: w290 -> [_ _]
                      frame False {
                      }
                      frame True {
                        n149 = Unbundle By Name(w301) -> ("Ping Channel"=w300:T16, "Echo Channel"=w299:T16)
                        n150 = Format Into String(format string="Ping %s; Echo %s", w300, w299) -> (resulting string=w303:string)  [unwired: 2 in, 1 out]
                        n151 = call <vilib>:"NT Write String.vi"("value"=w303, "name"=w302) -> ()  [unwired: 9 in, 1 out]
                      }
                    }
                  }
                  frame 1 {
                    # "I2C"
                    n152 = call-poly <vilib>:"WPI_UltrasonicRefNum Registry Get.vi"("refnum name"=w315) -> ("SonarSRF08_I2C_DevRef"=w309:T36)  [unwired: 9 in, 1 out]
                    n153 = Concatenate Strings(w314, w315, w311) -> (w308:string)
                    n154 = Concatenate Strings(w314, w315, w312) -> (w310:string)
                    n155 = call-poly <vilib>:"WPI_UltrasonicGetRange.vi"("SonarSRF08_I2C_DevRef"=w309) -> ("Light Sensor"=w305:u8, "Distance"=w306:u16)  [unwired: 7 in, 2 out]
                    n156 = Build Array(w306, w305) -> (w304:u16[])
                    n157 = call-poly <vilib>:"NT Write Value.vi"("value"=w304, "name"=w308) -> ("error out"=w307:errorcluster)  [unwired: 9 in]
                    n158 = case shown="True" w313 {
                      tunnel: w310 -> [_ w321]
                      tunnel: w309 -> [_ w319]
                      tunnel: w307 -> [_ _]
                      frame False {
                      }
                      frame True {
                        n159 = Unbundle(w319) -> ("I2CDevRef"=w318:T37)
                        n160 = Unbundle(w318) -> ("Device Address"=w316:u8, "I2C Bus"=w317:T27)  [unwired: 2 out]
                        n161 = Format Into String(format string="%s, addr %d", w317, w316) -> (resulting string=w322:string)  [unwired: 2 in, 1 out]
                        n162 = call <vilib>:"NT Write String.vi"("value"=w322, "name"=w321) -> ()  [unwired: 9 in, 1 out]
                      }
                    }
                  }
                  frame 2 {
                    # "I2C"
                    n163 = call-poly <vilib>:"WPI_UltrasonicRefNum Registry Get.vi"("refnum name"=w332) -> ("SonarMB1010DigitalDevRef"=w326:T38)  [unwired: 9 in, 1 out]
                    n164 = Concatenate Strings(w331, w332, w328) -> (w325:string)
                    n165 = Concatenate Strings(w331, w332, w329) -> (w327:string)
                    n166 = call-poly <vilib>:"WPI_UltrasonicGetRange.vi"("SonarMB1010DigitalDevRef"=w326) -> ("Distance"=w323:dbl)  [unwired: 8 in, 2 out]
                    n167 = call-poly <vilib>:"NT Write Value.vi"("value"=w323, "name"=w325) -> ("error out"=w324:errorcluster)  [unwired: 9 in]
                    n168 = case shown="True" w330 {
                      tunnel: w327 -> [_ w338]
                      tunnel: w326 -> [_ w336]
                      tunnel: w324 -> [_ _]
                      frame False {
                      }
                      frame True {
                        n169 = Unbundle(w336) -> ("CounterDevRef"=w335:T32, "Scaling factor (s/in)"=w333:dbl)
                        n170 = Unbundle(w335) -> ("CntIndex"=w334:T33)  [unwired: 1 out]
                        n171 = Format Into String(format string="%s, scale %f", w334, w333) -> (resulting string=w339:string)  [unwired: 2 in, 1 out]
                        n172 = call <vilib>:"NT Write String.vi"("value"=w339, "name"=w338) -> ()  [unwired: 9 in, 1 out]
                      }
                    }
                  }
                  frame 3 {
                    # "I2C"
                    n173 = call-poly <vilib>:"WPI_UltrasonicRefNum Registry Get.vi"("refnum name"=w349) -> ("SonarMB1010AnalogDevRef"=w343:T39)  [unwired: 9 in, 1 out]
                    n174 = Concatenate Strings(w348, w349, w345) -> (w342:string)
                    n175 = Concatenate Strings(w348, w349, w346) -> (w344:string)
                    n176 = call-poly <vilib>:"WPI_UltrasonicGetRange.vi"("SonarMB1010AnalogDevRef"=w343) -> ("Distance"=w340:dbl)  [unwired: 8 in, 2 out]
                    n177 = call-poly <vilib>:"NT Write Value.vi"("value"=w340, "name"=w342) -> ("error out"=w341:errorcluster)  [unwired: 9 in]
                    n178 = case shown="True" w347 {
                      tunnel: w344 -> [_ w356]
                      tunnel: w343 -> [_ w354]
                      tunnel: w341 -> [_ _]
                      frame False {
                      }
                      frame True {
                        n179 = Unbundle(w354) -> ("AIDeviceRef"=w353:T40, "Scaling factor (V/in)"=w351:dbl, "Average Bits"=w350:u8)
                        n180 = Unbundle(w353) -> ("Analog Channel"=w352:T26)  [unwired: 1 out]
                        n181 = Format Into String(format string="%s, scale %f, avg %d", w352, w351, w350) -> (resulting string=w357:string)  [unwired: 2 in, 1 out]
                        n182 = call <vilib>:"NT Write String.vi"("value"=w357, "name"=w356) -> ()  [unwired: 9 in, 1 out]
                      }
                    }
                  }
                }
              }
            }
          }
          frame "Digital In" {
            n183 = call <vilib>:"WPI_GetSetVariantRefNum.vi"("Operation"=w358, "refnum name"="Digital In:") -> ("names"=w359:string[])  [unwired: 7 in, 2 out]
            n184 = for {
              tunnel: w359 -> [w367] mode=indexing
              tunnel: w362 -> [w368]
              tunnel: w361 -> [w366]
              n185 = Concatenate Strings(w366, w367, "/Value") -> (w371:string)
              n186 = Concatenate Strings(w366, w367, "/Info") -> (w365:string)
              n187 = call <vilib>:"WPI_DigitalInputRefNum Registry Get.vi"("refnum name"=w367) -> ("DigitalInputDevRef"=w364:T41)  [unwired: 9 in, 1 out]
              n188 = call <vilib>:"WPI_DigitalInputGetValue.vi"("DigitalInputDevRef"=w364) -> ("Value"=w370:bool)  [unwired: 8 in, 2 out]
              n189 = call <vilib>:"NT Write Boolean.vi"("value"=w370, "name"=w371) -> ("error out"=w363:errorcluster)  [unwired: 9 in]
              n190 = case shown="True" w368 {
                tunnel: w365 -> [_ w373]
                tunnel: w364 -> [_ w374]
                tunnel: w363 -> [_ _]
                frame False {
                }
                frame True {
                  n191 = call <vilib>:"WPI_DigitalInputPublishInfo.vi"("Name"=w373, "DigitalInputDevRef"=w374) -> ()  [unwired: 10 in]
                }
              }
            }
          }
          frame "Switch" {
            n192 = call <vilib>:"WPI_GetSetVariantRefNum.vi"("Operation"=w375, "refnum name"="Switch:") -> ("names"=w376:string[])  [unwired: 7 in, 2 out]
            n193 = for {
              tunnel: w376 -> [w382] mode=indexing
              tunnel: w379 -> [w386]
              tunnel: w378 -> [w385]
              n194 = call <vilib>:"WPI_SwitchRefNum Registry Get.vi"("refnum name"=w382) -> ("SwitchDevRef"=w381:T42)  [unwired: 9 in, 1 out]
              n195 = Concatenate Strings(w385, w382, "/Value") -> (w388:string)
              n196 = Concatenate Strings(w385, w382, "/Info") -> (w384:string)
              n197 = Unbundle(w381) -> ("CntIndex"=w380:T33)  [unwired: 3 out]
              n198 = case shown="Default" w380 {
                tunnel: w388 -> [w390 w397]
                tunnel: [w391 w396] -> w383
                tunnel: w381 -> [w393 w394]
                frame Default {
                  n199 = call <vilib>:"WPI_SwitchGetCount.vi"("SwitchDevRef"=w393) -> ("Switch Pressed Count"=w392:i32)  [unwired: 8 in, 2 out]
                  n200 = call-poly <vilib>:"NT Write Value.vi"("value"=w392, "name"=w390) -> ("error out"=w391:errorcluster)  [unwired: 9 in]
                }
                frame "Invalid" {
                  n201 = call <vilib>:"WPI_SwitchGetLimitValue.vi"("SwitchDevRef"=w394) -> ("Switch Pressed"=w395:bool)  [unwired: 8 in, 2 out]
                  n202 = call <vilib>:"NT Write Boolean.vi"("value"=w395, "name"=w397) -> ("error out"=w396:errorcluster)  [unwired: 9 in]
                }
              }
              n203 = case shown="True" w386 {
                tunnel: w384 -> [_ w399]
                tunnel: w381 -> [_ w398]
                tunnel: w383 -> [_ _]
                frame False {
                }
                frame True {
                  n204 = call <vilib>:"WPI_SwitchPublishInfo.vi"("Name"=w399, "SwitchDevRef"=w398) -> ()  [unwired: 10 in]
                }
              }
            }
          }
          frame "Encoder" {
            n205 = call <vilib>:"WPI_GetSetVariantRefNum.vi"("Operation"=w400, "refnum name"="Encoder:") -> ("names"=w401:string[])  [unwired: 7 in, 2 out]
            n206 = for {
              tunnel: w401 -> [w407] mode=indexing
              tunnel: w404 -> [w416]
              tunnel: w403 -> [w408]
              n207 = Concatenate Strings(w408, w407, "/Distance") -> (w413:string)
              n208 = Concatenate Strings(w408, w407, "/Rate") -> (w410:string)
              n209 = Concatenate Strings(w408, w407, "/Info") -> (w415:string)
              n210 = call <vilib>:"WPI_EncoderRefNum Registry Get.vi"("refnum name"=w407) -> ("EncoderDevRef"=w414:T43)  [unwired: 9 in, 1 out]
              n211 = call <vilib>:"WPI_EncoderGet.vi"("EncoderDevRef"=w414) -> ("Distance"=w412:dbl, "Rate"=w409:dbl)  [unwired: 5 in, 4 out]
              n212 = call <vilib>:"NT Write Number.vi"("value"=w412, "name"=w413) -> ("error out"=w406:errorcluster)  [unwired: 9 in]
              n213 = call <vilib>:"NT Write Number.vi"("error in"=w406, "value"=w409, "name"=w410) -> ("error out"=w405:errorcluster)  [unwired: 8 in]
              n214 = case shown="True" w416 {
                tunnel: w415 -> [_ w422]
                tunnel: w414 -> [_ w419]
                tunnel: w405 -> [_ _]
                frame False {
                }
                frame True {
                  n215 = Unbundle(w419) -> ("EncoderIndex"=w420:T44, "CounterIndex"=w425:T33, "Decoding Type"=w421:T45)  [unwired: 2 out]
                  n216 = Format Into String(format string="%s, %s, %s", w421, w420, w425) -> (resulting string=w423:string)  [unwired: 2 in, 1 out]
                  n217 = call <vilib>:"NT Write String.vi"("value"=w423, "name"=w422) -> ()  [unwired: 9 in, 1 out]
                }
              }
            }
          }
          frame "Digital Out" {
            n218 = call <vilib>:"WPI_GetSetVariantRefNum.vi"("Operation"=w426, "refnum name"="Digital Out:") -> ("names"=w427:string[])  [unwired: 7 in, 2 out]
            n219 = for {
              tunnel: w427 -> [w434] mode=indexing
              tunnel: w430 -> [w436]
              tunnel: w429 -> [w433]
              n220 = call <vilib>:"WPI_DigitalOutputRefNum Registry Get.vi"("refnum name"=w434) -> ("DigitalOutputDevRef"=w431:T46)  [unwired: 9 in, 1 out]
              n221 = Concatenate Strings(w433, w434, "/Value  **") -> (w437:string)
              n222 = Concatenate Strings(w433, w434, "/Info") -> (w432:string)
              n223 = case shown="True" w436 {
                tunnel: w437 -> [w441 w448]
                tunnel: w431 -> [w442 w445]
                tunnel: w432 -> [_ w449]
                frame False {
                  n224 = call <vilib>:"NT Read Number.vi"("name"=w441) -> ("value"=w440:dbl)  [unwired: 8 in, 2 out]
                  n225 = Not Equal To 0?(x=w440) -> (x != 0?=w439:bool)
                  n226 = call <vilib>:"WPI_DigitalOutputSetValue.vi"("Value"=w439, "DigitalOutputDevRef"=w442) -> ()  [unwired: 8 in, 2 out]
                }
                frame True {
                  n227 = Unbundle By Name(w445) -> ("DIO Channel"=w446:T16)
                  n228 = call <vilib>:"NT Write Number.vi"("value"=0, "name"=w448) -> ("error out"=w444:errorcluster)  [unwired: 9 in]
                  n229 = call <vilib>:"WPI_DigitalOutputSetValue.vi"("error in (no error)"=w444, "Value"=FALSE, "DigitalOutputDevRef"=w445) -> ("error out"=w443:errorcluster)  [unwired: 7 in, 1 out]
                  n230 = Format Into String(format string="%s", w446) -> (resulting string=w451:string)  [unwired: 2 in, 1 out]
                  n231 = call <vilib>:"NT Write String.vi"("error in"=w443, "value"=w451, "name"=w449) -> ()  [unwired: 8 in, 1 out]
                }
              }
            }
          }
          frame "Analog Out" {
            n232 = call <vilib>:"WPI_GetSetVariantRefNum.vi"("Operation"=w453, "refnum name"="Analog Out:") -> ("names"=w454:string[])  [unwired: 7 in, 2 out]
            n233 = for {
              tunnel: w454 -> [w459] mode=indexing
              tunnel: w457 -> [w463]
              tunnel: w456 -> [w461]
              n234 = call <vilib>:"WPI_AnalogOutputRefNum Registry Get.vi"("refnum name"=w459) -> ("AODeviceRef"=w458:T47)  [unwired: 9 in, 1 out]
              n235 = Concatenate Strings(w461, w459, "/Value  **") -> (w464:string)
              n236 = Concatenate Strings(w461, w459, "/Info") -> (w460:string)
              n237 = case shown="False" w463 {
                tunnel: w464 -> [w468 w475]
                tunnel: w458 -> [w467 w472]
                tunnel: w460 -> [_ w476]
                frame False {
                  n238 = call <vilib>:"NT Read Number.vi"("name"=w468) -> ("value"=w466:dbl)  [unwired: 8 in, 2 out]
                  n239 = call <vilib>:"WPI_AnalogOutputSetVoltage.vi"("Voltage"=w466, "AODeviceRef"=w467) -> ()  [unwired: 8 in, 2 out]
                }
                frame True {
                  n240 = Unbundle By Name(w472) -> ("AO Channel"=w473:T48)
                  n241 = call <vilib>:"NT Write Number.vi"("value"=0, "name"=w475) -> ("error out"=w470:errorcluster)  [unwired: 9 in]
                  n242 = call <vilib>:"WPI_AnalogOutputSetVoltage.vi"("error in (no error)"=w470, "Voltage"=0.0, "AODeviceRef"=w472) -> ("error out"=w469:errorcluster)  [unwired: 7 in, 1 out]
                  n243 = Format Into String(format string="%s", w473) -> (resulting string=w478:string)  [unwired: 2 in, 1 out]
                  n244 = call <vilib>:"NT Write String.vi"("error in"=w469, "value"=w478, "name"=w476) -> ()  [unwired: 8 in, 1 out]
                }
              }
            }
          }
          frame "PWM" {
            n245 = call <vilib>:"WPI_GetSetVariantRefNum.vi"("Operation"=w479, "refnum name"="PWM:") -> ("names"=w480:string[])  [unwired: 7 in, 2 out]
            n246 = for {
              tunnel: w480 -> [w487] mode=indexing
              tunnel: w483 -> [w490]
              tunnel: w482 -> [w486]
              n247 = call <vilib>:"WPI_PWMRefNum Registry Get.vi"("refnum name"=w487) -> ("PWMDeviceRef"=w484:T49)  [unwired: 9 in, 1 out]
              n248 = Concatenate Strings(w486, w487, "/Value  **") -> (w491:string)
              n249 = Concatenate Strings(w486, w487, "/Info") -> (w485:string)
              n250 = case shown="False" w490 {
                tunnel: w491 -> [w494 w502]
                tunnel: [w493 w501] -> w489
                tunnel: w484 -> [_ w497]
                tunnel: w485 -> [_ w498]
                frame False {
                  n251 = call <vilib>:"NT Read Number.vi"("name"=w494) -> ("value"=w493:dbl)  [unwired: 8 in, 2 out]
                }
                frame True {
                  w501 = u8 0 ("Value")
                  n252 = Unbundle By Name(w497) -> ("PWM Channel"=w496:T14)
                  n253 = call <vilib>:"NT Write Number.vi"("value"=w501, "name"=w502) -> ("error out"=w495:errorcluster)  [unwired: 9 in]
                  n254 = Format Into String(format string=" %s", w496) -> (resulting string=w500:string)  [unwired: 2 in, 1 out]
                  n255 = call <vilib>:"NT Write String.vi"("error in"=w495, "value"=w500, "name"=w498) -> ()  [unwired: 8 in, 1 out]
                }
              }
              n256 = call <vilib>:"WPI_PWMSetValue.vi"("Value"=w489, "PWMDeviceRef"=w484) -> ()  [unwired: 8 in, 2 out]
            }
          }
          frame "Analog In" {
            n257 = call <vilib>:"WPI_GetSetVariantRefNum.vi"("Operation"=w503, "refnum name"="Analog In:") -> ("names"=w504:string[])  [unwired: 7 in, 2 out]
            n258 = for {
              tunnel: w504 -> [w512] mode=indexing
              tunnel: w507 -> [w514]
              tunnel: w506 -> [w511]
              n259 = call <vilib>:"WPI_AnalogChannelRefNum Registry Get.vi"("refnum name"=w512) -> ("AIDeviceRef"=w509:T40)  [unwired: 9 in, 1 out]
              n260 = Concatenate Strings(w511, w512, "/Voltage") -> (w516:string)
              n261 = Concatenate Strings(w511, w512, "/Info") -> (w510:string)
              n262 = call <vilib>:"WPI_AnalogChannelGetVoltage.vi"("AIDeviceRef"=w509) -> ("Voltage"=w515:dbl)  [unwired: 8 in, 2 out]
              n263 = call <vilib>:"NT Write Number.vi"("value"=w515, "name"=w516) -> ("error out"=w508:errorcluster)  [unwired: 9 in]
              n264 = case shown="True" w514 {
                tunnel: w510 -> [_ w520]
                tunnel: w509 -> [_ w518]
                tunnel: w508 -> [_ _]
                frame False {
                }
                frame True {
                  n265 = Unbundle By Name(w518) -> ("Analog Channel"=w519:T26)
                  n266 = Format Into String(format string="%s", w519) -> (resulting string=w521:string)  [unwired: 2 in, 1 out]
                  n267 = call <vilib>:"NT Write String.vi"("value"=w521, "name"=w520) -> ()  [unwired: 9 in, 1 out]
                }
              }
            }
          }
          frame "Potentiometer" {
            n268 = call <vilib>:"WPI_GetSetVariantRefNum.vi"("Operation"=w523, "refnum name"="Potentiometer:") -> ("names"=w524:string[])  [unwired: 7 in, 2 out]
            n269 = for {
              tunnel: w524 -> [w530] mode=indexing
              tunnel: w527 -> [w535]
              tunnel: w526 -> [w533]
              n270 = call <vilib>:"WPI_PotentiometerRefNum Registry Get.vi"("refnum name"=w530) -> ("PotDevRef"=w529:T50)  [unwired: 9 in, 1 out]
              n271 = Concatenate Strings(w533, w530, "/Value") -> (w536:string)
              n272 = Concatenate Strings(w533, w530, "/Info") -> (w532:string)
              n273 = call <vilib>:"WPI_PotentiometerGetTestValue.vi"("PotDevRef"=w529) -> ("Test Value"=w528:dbl)  [unwired: 8 in, 2 out]
              n274 = call <vilib>:"NT Write Number.vi"("value"=w528, "name"=w536) -> ("error out"=w531:errorcluster)  [unwired: 9 in]
              n275 = case shown="True" w535 {
                tunnel: w532 -> [_ w544]
                tunnel: w529 -> [_ w542]
                tunnel: w531 -> [_ _]
                frame False {
                }
                frame True {
                  n276 = Unbundle By Name(w542) -> ("Analog Channel"=w543:T26, "Invert Output"=w541:bool)
                  n277 = Select(t="(inverted)" ("format string"), s=w541, f="" ("format string")) -> (s? t:f=w538:string)
                  n278 = Format Into String(format string="%s, %s", w543, w538) -> (resulting string=w545:string)  [unwired: 2 in, 1 out]
                  n279 = call <vilib>:"NT Write String.vi"("value"=w545, "name"=w544) -> ()  [unwired: 9 in, 1 out]
                }
              }
            }
          }
          frame "Camera" {
            n280 = call <vilib>:"WPI_GetSetVariantRefNum.vi"("Operation"=w547, "refnum name"="Camera:") -> ("names"=w548:string[])  [unwired: 7 in, 2 out]
            n281 = for {
              tunnel: w548 -> [w555] mode=indexing
              tunnel: w551 -> [w557]
              tunnel: w550 -> [w556]
              n282 = call <vilib>:"WPI_CameraRefNum Registry Get.vi"("refnum name"=w555) -> ("CameraDevRef"=w554:T51)  [unwired: 9 in, 1 out]
              n283 = Unbundle By Name(w554) -> ("Camera Address"=w553:string)
              n284 = call <vilib>:"WPI_CameraIsSimulated.vi"("Camera Address"=w553) -> ("Simulated"=w552:bool)  [unwired: 10 in]
              n285 = case shown="False" w552 {
                tunnel: w557 -> [w561 _]
                tunnel: w556 -> [w560 _]
                tunnel: w555 -> [w559 _]
                tunnel: w554 -> [w558 _]
                frame False {
                  n286 = case shown="True" w561 {
                    tunnel: w558 -> [w564 w567]
                    tunnel: w560 -> [w563 w566]
                    tunnel: w559 -> [w562 w565]
                    frame False {
                      n287 = call <vilib>:"WPI_CameraUpdate Settings.vi"("Name"=w562, "Table"=w563, "CameraDevRef"=w564) -> ()  [unwired: 9 in]
                    }
                    frame True {
                      n288 = call <vilib>:"WPI_CameraPublish Settings.vi"("Name"=w565, "Table"=w566, "CameraDevRef"=w567) -> ()  [unwired: 9 in]
                    }
                  }
                }
                frame True {
                  # "ignore for simulation"
                }
              }
            }
          }
          frame "Serial" {
            n289 = case shown="True" w568 {
              tunnel: w570 -> [_ w576]
              tunnel: w569 -> [_ w573]
              frame False {
              }
              frame True {
                n290 = call <vilib>:"WPI_GetSetVariantRefNum.vi"("Operation"=w573, "refnum name"="Serial:") -> ("names"=w574:string[])  [unwired: 7 in, 2 out]
                n291 = for {
                  tunnel: w574 -> [w597] mode=indexing
                  tunnel: w576 -> [w596]
                  tunnel: refnum<visa-resource-name> "ASRL1::INSTR" ("VISA resource name") -> [w599]
                  tunnel: "%s (baud %d, data %d, parity %s, stop %s, flow %s)" -> [w586]
                  n292 = call <vilib>:"WPI_SerialPortRefNum Registry Get.vi"("refnum name"=w597) -> ("SerialPortRef"=w600:T52)  [unwired: 9 in, 1 out]
                  n293 = Concatenate Strings(w596, w597, "/Info") -> (w595:string)
                  n294 = Unbundle(w600) -> ("Serial Port Name"=w590:refnum<visa-resource-name>)  [unwired: 1 out]
                  n295 = property class="Instr"(reference=w590) -> ("Baud"=w588:u32, "Data Bits"=w587:u16, "Parity"=w584:u16, "Stop Bits"=w582:u16, "Flow Cntrl"=w579:u16)  [unwired: 1 in, 2 out]
                  n296 = Equal?(x=w599, y=w590) -> (x = y?=w594:bool)
                  n297 = Select(t="Onboard", s=w594, f="MXP") -> (s? t:f=w591:string)
                  n298 = Type Cast(type=enum16{"1.0", "1.5", "2.0"}."1.0" ("Stop Bits"), x=w582) -> (*(type *) &x=w580:enum16{"1.0", "1.5", "2.0"})
                  n299 = Type Cast(type=T5."None" ("Flow Control"), x=w579) -> (*(type *) &x=w577:T5)
                  n300 = Type Cast(type=enum16{"None", "Odd", "Even", "Mark", "Space"}."None" ("Parity"), x=w584) -> (*(type *) &x=w583:enum16{"None", "Odd", "Even", "Mark", "Space"})
                  n301 = Format Into String(format string=w586, w591, w588, w587, w583, w580, w577) -> (resulting string=w589:string)  [unwired: 2 in, 1 out]
                  n302 = call <vilib>:"NT Write String.vi"("value"=w589, "name"=w595) -> ()  [unwired: 9 in, 1 out]
                }
              }
            }
          }
          frame "I2C" {
            n303 = case shown="True" w601 {
              tunnel: w603 -> [_ w607]
              tunnel: w602 -> [_ w604]
              frame False {
              }
              frame True {
                n304 = call <vilib>:"WPI_GetSetVariantRefNum.vi"("Operation"=w604, "refnum name"="I2C:") -> ("names"=w605:string[])  [unwired: 7 in, 2 out]
                n305 = for {
                  tunnel: w605 -> [w612] mode=indexing
                  tunnel: w607 -> [w615]
                  n306 = call <vilib>:"WPI_I2CRefNum Registry Get.vi"("refnum name"=w612) -> ("I2CDevRef"=w611:T37)  [unwired: 9 in, 1 out]
                  n307 = Concatenate Strings(w615, w612, "/Info") -> (w614:string)
                  n308 = Unbundle(w611) -> ("Device Address"=w609:u8, "I2C Bus"=w610:T27)  [unwired: 2 out]
                  n309 = Format Into String(format string="%s, addr %d,", w610, w609) -> (resulting string=w613:string)  [unwired: 2 in, 1 out]
                  n310 = call <vilib>:"NT Write String.vi"("value"=w613, "name"=w614) -> ()  [unwired: 9 in, 1 out]
                }
              }
            }
          }
          frame "SPI" {
            n311 = case shown="True" w617 {
              tunnel: w619 -> [_ w623]
              tunnel: w618 -> [_ w620]
              frame False {
              }
              frame True {
                n312 = call <vilib>:"WPI_GetSetVariantRefNum.vi"("Operation"=w620, "refnum name"="SPI:") -> ("names"=w621:string[])  [unwired: 7 in, 2 out]
                n313 = for {
                  tunnel: w621 -> [w626] mode=indexing
                  tunnel: w623 -> [w630]
                  n314 = call <vilib>:"WPI_SPIRefNum Registry Get.vi"("refnum name"=w626) -> ("SPIDevRef"=w625:T53)  [unwired: 9 in, 1 out]
                  n315 = Concatenate Strings(w630, w626, "/Info") -> (w629:string)
                  n316 = Unbundle(w625) -> ("SPI Bus"=w624:T28)  [unwired: 2 out]
                  n317 = Format Into String(format string="%s", w624) -> (resulting string=w628:string)  [unwired: 2 in, 1 out]
                  n318 = call <vilib>:"NT Write String.vi"("value"=w628, "name"=w629) -> ()  [unwired: 9 in, 1 out]
                }
              }
            }
          }
        }
      }
    }
  }
